vi "Start Acquisition.vi"(8 "error in (no error)":errorcluster, 11 "SPARC4_GEI in":refnum<class "SPARC4_GEI.lvclass">) -> (0 "error out":errorcluster, 3 "SPARC4_GEI out":refnum<class "SPARC4_GEI.lvclass">)   [LabVIEW 2018, in "SPARC4_GEI.lvclass"]
uses:
  SPARC4_GEI.lvclass
  SPARC4_GEI.lvclass/SPARC4_GEI.ctl
  Channel GUI/Channel GEI.lvclass
  TCS/TCS.lvclass
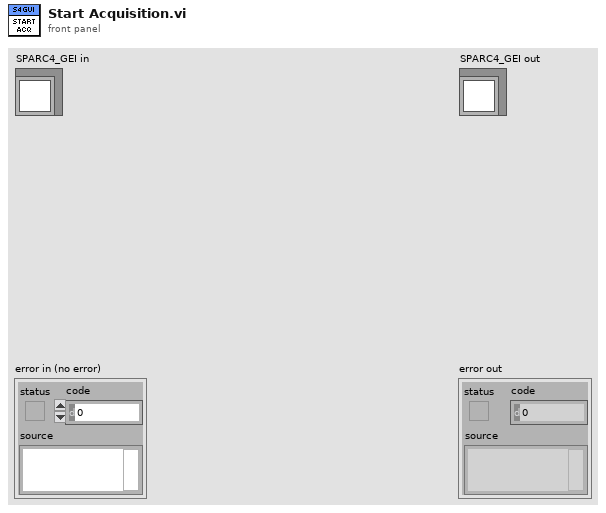
[diagram p1: front panel]
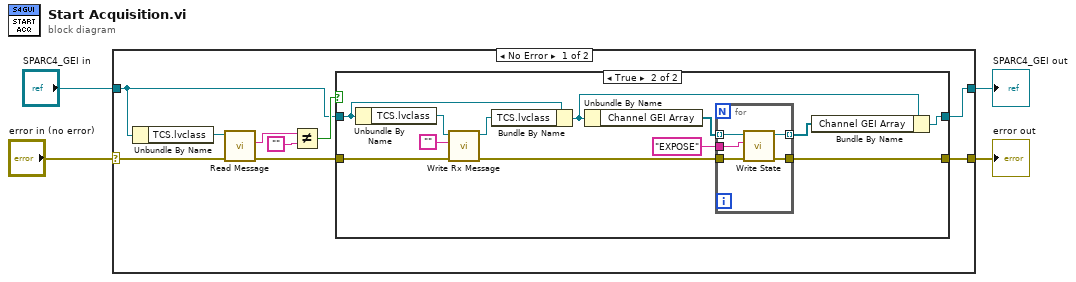
[diagram p0: block diagram]
diagram:
  n1 = case shown="No Error" "error in (no error)" {
    selector: "error in (no error)" -> [w7 w34]
    tunnel: [w11 w34] -> w3
    tunnel: [w9 w33] -> w2
    tunnel: "SPARC4_GEI in" -> [w10 w33]
    frame No Error {
      n2 = Unbundle By Name(w10) -> ("TCS.lvclass"=w8:refnum<class "TCS.lvclass">)
      n3 = call "Read Message.vi"("error in (no error)"=w7, "TCS in"=w8) -> ("error out"=w5:errorcluster, "Rx Message"=w6:string)  [unwired: 7 in, 1 out]
      n4 = Not Equal?(x=w6, y="") -> (x != y?=w12:bool)
      n5 = case shown="True" w12 {
        tunnel: w5 -> [w14 w20]
        tunnel: [w14 w27] -> w11
        tunnel: w10 -> [w15 w21]
        tunnel: [w15 w23] -> w9
        frame False {
        }
        frame True {
          n6 = Unbundle By Name(w21) -> ("TCS.lvclass"=w17:refnum<class "TCS.lvclass">)
          n7 = call "Write Rx Message.vi"("error in (no error)"=w20, "Rx Message"="", "TCS in"=w17) -> ("error out"=w19:errorcluster, "TCS out"=w18:refnum<class "TCS.lvclass">)  [unwired: 7 in]
          n8 = Bundle By Name(cluster=w21, "TCS.lvclass"=w18) -> (w22:refnum<class "SPARC4_GEI.lvclass">)
          n9 = Unbundle By Name(w22) -> ("Channel GEI Array"=w25:refnum<class "Channel GEI.lvclass">[])
          n10 = for {
            tunnel: [w32] -> w24 mode=indexing
            tunnel: [w31] -> w27
            tunnel: "EXPOSE" -> [w30]
            tunnel: w25 -> [w29] mode=indexing
            tunnel: w19 -> [w28]
            n11 = call "Write State.vi"("error in (no error)"=w28, "State"=w30, "Channel GEI in"=w29) -> ("error out"=w31:errorcluster, "Channel GEI out"=w32:refnum<class "Channel GEI.lvclass">)  [unwired: 7 in]
          }
          n12 = Bundle By Name(cluster=w22, "Channel GEI Array"=w24) -> (w23:refnum<class "SPARC4_GEI.lvclass">)
        }
      }
    }
    frame Error {
    }
  }
  "error out" <- w3
  "SPARC4_GEI out" <- w2
